vi "ReversedEngineering FindStateIndexToJumpTo.vi"(1 "String":string, 2 "Array":string[](array[string])) -> (0 "index of element":i32)   [LabVIEW 2014]
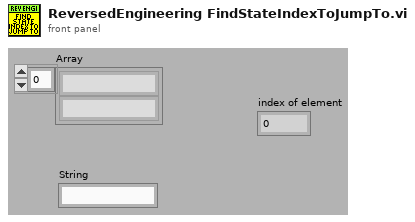
[diagram p1: front panel]
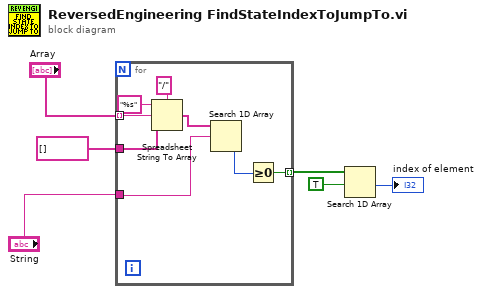
[diagram p0: block diagram]
diagram:
  n1 = for {
    tunnel: "Array" -> [w14] mode=indexing
    tunnel: "String" -> [w9]
    tunnel: string[] [] ("Array") -> [w11]
    tunnel: [w7] -> w3 mode=indexing
    n2 = Spreadsheet String To Array(delimiter (Tab)="/", format string="%s", spreadsheet string=w14, array type (2D Dbl)=w11) -> (array=w10:string[])
    n3 = Search 1D Array(1D array=w10, element=w9) -> (index of element=w8:i32)  [unwired: 1 out]
    n4 = Greater Or Equal To 0?(x=w8) -> (x >= 0?=w7:bool)
  }
  n5 = Search 1D Array(1D array=w3, element=TRUE) -> (index of element=→"index of element":i32)  [unwired: 1 out]
